vi "Three Button Dialog CORE.vi"(4 "Allow user to close window? (TRUE)":bool=TRUE, 5 "Justify Message (Left)":enum16{"Left", "Center", "Right"}(ring), 6 "Keyboard Shortcuts (Left is <Enter>)":T1={"Left Button Key Shortcut"={"Control"=FALSE, "Shift"=FALSE, "Key"="<Enter>"}, "Center Button Key Shortcut"={"Control"=FALSE, "Shift"=FALSE, "Key"=""}, "Right Button Key Shortcut"={"Control"=FALSE, "Shift"=FALSE, "Key"=""}}, 7 "Window Title (\"\")":string, 8 "Right Button Text (\"Cancel\")":string="Cancel", 9 "Center Button Text (\"No\")":string="No", 10 "Left Button Text (\"Yes\")":string="Yes", 11 "message":string) -> (3 "Which Button?":T2(ring)=enum."Center Button")   [LabVIEW 2011]
doc: "Displays text in a dialog with three buttons. The output enum indicates which of the three buttons the user chose, or it indicates that the user closed the dialog without making any choice."
panel:
  in  "OK":string="OK"
  out "C-Message":string
  in  "Right Button":bool
  in  "Center Button":bool
  in  "Left Button":bool
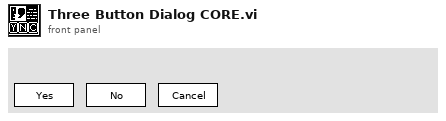
[diagram p1: front panel]
types:
  T1 = cluster{"Left Button Key Shortcut":cluster{"Control":bool, "Shift":bool, "Key":string}, "Center Button Key Shortcut":cluster{"Control":bool, "Shift":bool, "Key":string}, "Right Button Key Shortcut":cluster{"Control":bool, "Shift":bool, "Key":string}}
  T2 = enum16{"Left Button", "Center Button", "Right Button", "Window Close"}
  T3 = cluster{"left":i16, "top":i16, "right":i16, "bottom":i16}
  T4 = cluster{"Control":bool, "Shift":bool, "Key":string}
  T5 = cluster{bool, "Control":bool, "Shift":bool, "Key":string}
  T6 = typedef "LVRectTypeDef.ctl" = cluster{"left":i16, "top":i16, "right":i16, "bottom":i16}
  T7 = typedef "LVBoundsTypeDef.ctl" = cluster{"Width":u32, "Height":u32}
  T8 = typedef "LVPointTypeDef.ctl" = cluster{"Horizontal":i16, "Vertical":i16}
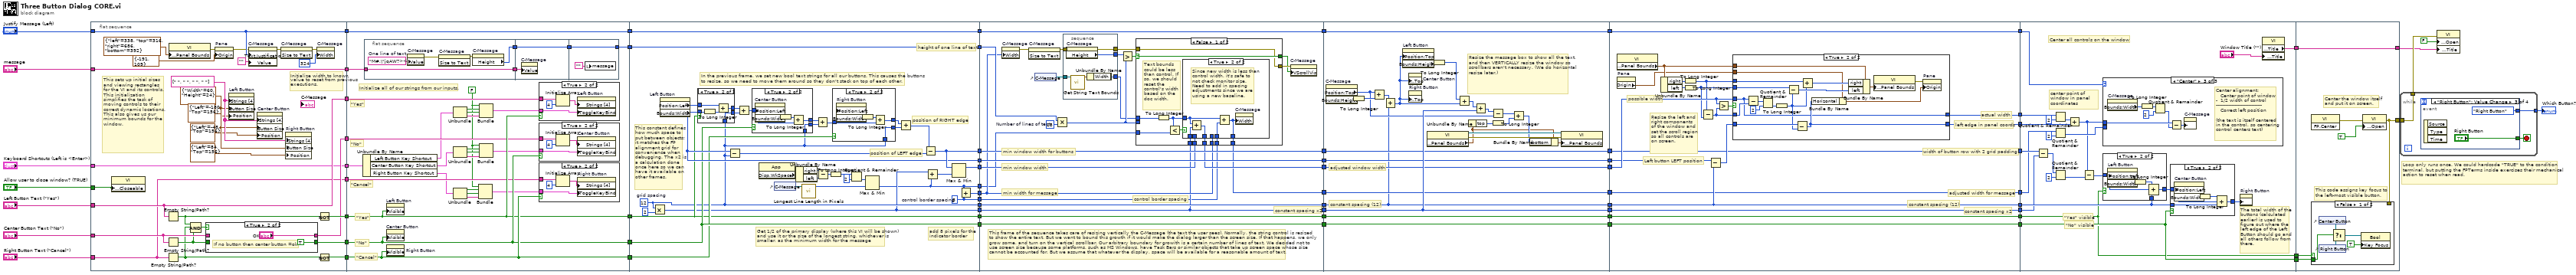
[diagram p0: block diagram]
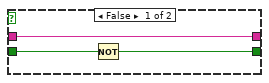
[diagram p2: hidden frame]
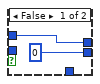
[diagram p6: hidden frame]
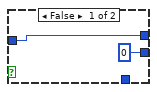
[diagram p7: hidden frame]
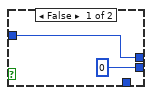
[diagram p8: hidden frame]
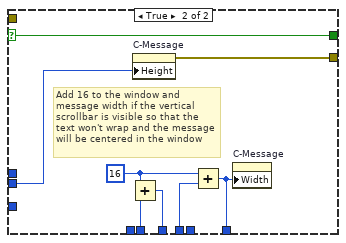
[diagram p10: hidden frame]
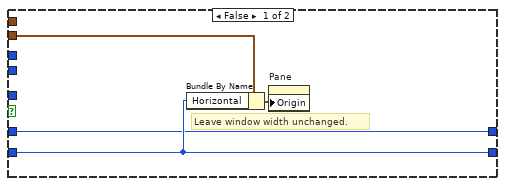
[diagram p11: hidden frame]
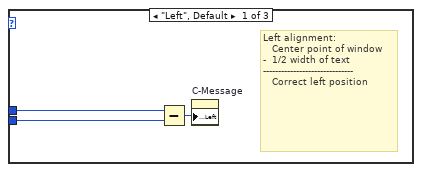
[diagram p12: hidden frame]
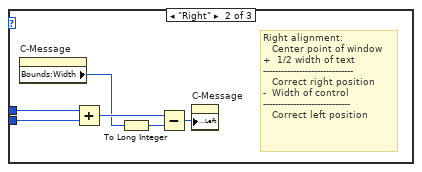
[diagram p13: hidden frame]
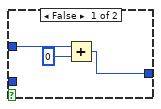
[diagram p14: hidden frame]
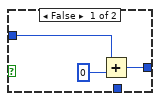
[diagram p15: hidden frame]
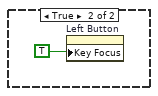
[diagram p16: hidden frame]
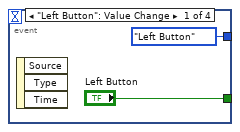
[diagram p17: hidden frame]
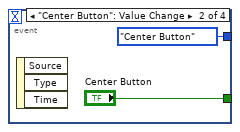
[diagram p18: hidden frame]
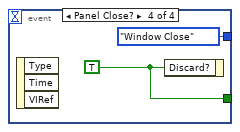
[diagram p19: hidden frame]
diagram:
  # "Loop only runs once. We could hardcode \"TRUE\" to the condition terminal, but putting the FPTerms inside exercises their mechanical action to reset when read."
  n1 = flat-sequence {
    tunnel: [w86] -> w14
    tunnel: [w88] -> w13
    tunnel: [w87] -> w12
    tunnel: [w82] -> w11
    tunnel: [w83] -> w10
    tunnel: [w80] -> w9
    tunnel: [w79] -> w8
    tunnel: "Left Button Text (\"Yes\")" -> [w82]
    tunnel: "Center Button Text (\"No\")" -> [w81]
    tunnel: "Right Button Text (\"Cancel\")" -> [w80]
    tunnel: "Justify Message (Left)" -> [w79]
    tunnel: "Keyboard Shortcuts (Left is <Enter>)" -> [w76]
    tunnel: [w76] -> w7
    tunnel: "message" -> [w75]
    tunnel: [w75] -> w6
    tunnel: "Allow user to close window? (TRUE)" -> [w74]
    tunnel: w14 -> [w130]
    tunnel: [w130] -> w64
    tunnel: w13 -> [w129]
    tunnel: [w129] -> w63
    tunnel: w12 -> [w128]
    tunnel: [w128] -> w62
    tunnel: w11 -> [w127]
    tunnel: w10 -> [w126]
    tunnel: w9 -> [w125]
    tunnel: w8 -> [w124]
    tunnel: [w124] -> w61
    tunnel: [w120] -> w60
    tunnel: w7 -> [w123]
    tunnel: w6 -> [w119]
    tunnel: [w185] -> w59
    tunnel: [w182] -> w58
    tunnel: [w181] -> w57
    tunnel: [w164] -> w56
    tunnel: [w163] -> w55
    tunnel: w64 -> [w174]
    tunnel: w63 -> [w176]
    tunnel: [w176] -> w54
    tunnel: w62 -> [w172]
    tunnel: [w172] -> w53
    tunnel: [w155] -> w52
    tunnel: w61 -> [w167]
    tunnel: [w167] -> w51
    tunnel: w60 -> [w166]
    tunnel: [w166] -> w50
    tunnel: [w153] -> w3
    tunnel: [w152] -> w2
    tunnel: w59 -> [w220]
    tunnel: [w219] -> w49
    tunnel: w58 -> [w226]
    tunnel: [w226] -> w48
    tunnel: w57 -> [w225]
    tunnel: [w225] -> w47
    tunnel: w56 -> [w224]
    tunnel: [w224] -> w46
    tunnel: w55 -> [w213]
    tunnel: [w213] -> w45
    tunnel: w54 -> [w223]
    tunnel: [w223] -> w44
    tunnel: w53 -> [w222]
    tunnel: [w222] -> w43
    tunnel: w52 -> [w214]
    tunnel: [w218] -> w42
    tunnel: w51 -> [w221]
    tunnel: [w221] -> w41
    tunnel: w50 -> [w216]
    tunnel: w3 -> [w212]
    tunnel: w2 -> [w211]
    tunnel: w49 -> [w275]
    tunnel: [w275] -> w40
    tunnel: w48 -> [w274]
    tunnel: [w274] -> w39
    tunnel: w47 -> [w273]
    tunnel: [w273] -> w38
    tunnel: w46 -> [w266]
    tunnel: [w266] -> w37
    tunnel: w45 -> [w283]
    tunnel: [w283] -> w36
    tunnel: w44 -> [w272]
    tunnel: [w272] -> w35
    tunnel: w43 -> [w271]
    tunnel: [w271] -> w34
    tunnel: w42 -> [w270]
    tunnel: [w270] -> w33
    tunnel: w41 -> [w269]
    tunnel: [w269] -> w32
    tunnel: w40 -> [w310]
    tunnel: [w305] -> w31
    tunnel: w39 -> [w298]
    tunnel: [w298] -> w30
    tunnel: w38 -> [w304]
    tunnel: w37 -> [w303]
    tunnel: [w303] -> w29
    tunnel: w36 -> [w297]
    tunnel: [w297] -> w28
    tunnel: [w301] -> w27
    tunnel: w35 -> [w296]
    tunnel: [w296] -> w26
    tunnel: w34 -> [w295]
    tunnel: [w295] -> w25
    tunnel: w33 -> [w292]
    tunnel: [w292] -> w24
    tunnel: w32 -> [w294]
    tunnel: [w294] -> w23
    tunnel: [w335] -> w22
    tunnel: w31 -> [w354]
    tunnel: w30 -> [w347]
    tunnel: w29 -> [w351]
    tunnel: w28 -> [w346]
    tunnel: w27 -> [w353]
    tunnel: w26 -> [w334]
    tunnel: w25 -> [w333]
    tunnel: w24 -> [w339]
    tunnel: w23 -> [w340]
    tunnel: [w334] -> w5
    tunnel: [w333] -> w4
    tunnel: [w388] -> w67
    tunnel: [w390] -> w65
    tunnel: w22 -> [w390]
    tunnel: w5 -> [w386]
    tunnel: w4 -> [w387]
    frame #0 {
      w96 = string[] [" ", " ", " ", " "] ("Strings [4]")
      w95 = cluster{"Width":u32, "Height":u32} {"Width"=60, "Height"=24} ("Button Size")
      # "Initialize width to known value to reset from previous executions."
      # "This sets up initial sizes and viewing rectangles\nfor the VI and its controls. This initialization\nsimplifies the task of moving controls to their\ncorrect dynamic locations. This also gives us our\nminimum bounds for the window."
      n2 = property class="VI"("Front Panel Window:Closeable"=w74) -> ()  [unwired: 2 in, 2 out]
      n3 = Empty String/Path?(string/path=w82) -> (empty?=w90:bool)
      n4 = Empty String/Path?(string/path=w81) -> (empty?=w78:bool)
      n5 = Empty String/Path?(string/path=w80) -> (empty?=w77:bool)
      n6 = property class="VI"("Front Panel Window:Panel Bounds"=T3 {"left"=338, "top"=316, "right"=686, "bottom"=392} ("Front Panel.PanelBounds")) -> (error out=w73:errorcluster)  [unwired: 2 in, 1 out]
      n7 = Compound Arithmetic op=AND(w90, w77, w78) -> (w89:bool)
      n8 = case shown="True" w89 {
        tunnel: w78 -> [w99 _]
        tunnel: [w98 TRUE] -> w88
        tunnel: w81 -> [w97 _]
        tunnel: [w97 "OK"] -> w83
        frame False {
          n9 = Not(x=w99) -> (.not. x?=w98:bool)
        }
        frame True {
          # "If no button then center button =ok"
        }
      }
      n10 = property on="Pane" class="Pane"(error in=w73, "Origin"=cluster{"Horizontal":i16, "Vertical":i16} {"Horizontal"=-191, "Vertical"=109} ("Front Panel.Origin")) -> (error out=w72:errorcluster)  [unwired: 1 in, 1 out]
      n11 = property on="Left Button" class="Bool"("Strings [4]"=w96, "Button Size"=w95, "Position"=cluster{"Left":i32, "Top":i32} {"Left"=-180, "Top"=156}) -> ()  [unwired: 2 in, 2 out]
      n12 = property on="C-Message" class="Str"(error in=w72, "Text.Justification"=w79, "Value"="") -> (error out=w91:errorcluster)  [unwired: 1 in, 1 out]
      n13 = property on="Center Button" class="Bool"("Strings [4]"=w96, "Button Size"=w95, "Position"=cluster{"Left":i32, "Top":i32} {"Left"=-48, "Top"=156}) -> ()  [unwired: 2 in, 2 out]
      n14 = invoke on="C-Message" class="Str" method="Size to Text"(error in=w91) -> (error out=w70:errorcluster)  [unwired: 2 in, 2 out]
      n15 = property on="Right Button" class="Bool"("Strings [4]"=w96, "Button Size"=w95, "Position"=cluster{"Left":i32, "Top":i32} {"Left"=84, "Top"=156}) -> ()  [unwired: 2 in, 2 out]
      n16 = property on="C-Message" class="Str"(error in=w70, "Width"=u32 324 ("Size:Width")) -> ()  [unwired: 1 in, 2 out]
      n17 = Not(x=w90) -> (.not. x?=w87:bool)
      n18 = Not(x=w77) -> (.not. x?=w86:bool)
    }
    frame #1 {
      w104 = FALSE
      # "\"Cancel\""
      # "\"No\""
      # "\"Yes\""
      # "\"Cancel\""
      # "\"No\""
      # "\"Yes\""
      # "Initialize all of our strings from our inputs."
      n19 = Unbundle By Name(w123) -> ("Left Button Key Shortcut"=w117:T4, "Center Button Key Shortcut"=w109:T4, "Right Button Key Shortcut"=w103:T4)
      n20 = flat-sequence {
        tunnel: [w132] -> w122
        tunnel: w119 -> [w131]
        tunnel: [w131] -> w118
        tunnel: w122 -> [w137]
        tunnel: [w137] -> w121
        tunnel: w118 -> [w136]
        tunnel: w121 -> [w138]
        tunnel: [w138] -> w120
        frame #0 {
          w135 = "M#,\"jqAW?><"  # One line of text
          n21 = property on="C-Message" class="Str"("Value"=w135) -> (error out=w133:errorcluster)  [unwired: 2 in, 1 out]
          n22 = invoke on="C-Message" class="Str" method="Size to Text"(error in=w133) -> (error out=w134:errorcluster)  [unwired: 2 in, 2 out]
          n23 = property on="C-Message" class="Str"(error in=w134) -> ("Height"=w132:u32)  [unwired: 1 in, 2 out]
        }
        frame #1 {
          n24 = property on="C-Message" class="Str"("Value"=w136) -> ()  [unwired: 2 in, 2 out]
        }
        frame #2 {
          n25 = local write "message"("") -> ()
        }
      }
      n26 = property on="Left Button" class="Bool"("Visible"=w128) -> ()  [unwired: 2 in, 2 out]
      n27 = property on="Center Button" class="Bool"("Visible"=w129) -> ()  [unwired: 2 in, 2 out]
      n28 = property on="Right Button" class="Bool"("Visible"=w130) -> ()  [unwired: 2 in, 2 out]
      n29 = Unbundle(w117) -> ("Control"=w116:bool, "Shift"=w115:bool, "Key"=w114:string)
      n30 = Unbundle(w109) -> ("Control"=w112:bool, "Shift"=w111:bool, "Key"=w110:string)
      n31 = Unbundle(w103) -> ("Control"=w107:bool, "Shift"=w106:bool, "Key"=w105:string)
      n32 = Bundle(w104, "Control"=w107, "Shift"=w106, "Key"=w105) -> (w102:T5)  [unwired: 1 out]
      n33 = Bundle(w104, "Control"=w116, "Shift"=w115, "Key"=w114) -> (w113:T5)  [unwired: 1 out]
      n34 = Bundle(w104, "Control"=w112, "Shift"=w111, "Key"=w110) -> (w108:T5)  [unwired: 1 out]
      n35 = case shown="True" w128 {
        tunnel: w127 -> [_ w149]
        tunnel: w113 -> [_ w148]
        frame False {
        }
        frame True {
          n36 = Initialize Array(w149, 4 ("dimension size")) -> (w151:string[])
          n37 = property on="Left Button" class="Bool"("Strings [4]"=w151, "ToggleKeyBind"=w148) -> ()  [unwired: 2 in, 2 out]
        }
      }
      n38 = case shown="True" w129 {
        tunnel: w108 -> [_ w145]
        tunnel: w126 -> [_ w144]
        frame False {
        }
        frame True {
          n39 = Initialize Array(w144, 4 ("dimension size")) -> (w147:string[])
          n40 = property on="Center Button" class="Bool"("Strings [4]"=w147, "ToggleKeyBind"=w145) -> ()  [unwired: 2 in, 2 out]
        }
      }
      n41 = case shown="True" w130 {
        tunnel: w102 -> [_ w141]
        tunnel: w125 -> [_ w140]
        frame False {
        }
        frame True {
          n42 = Initialize Array(w140, 4 ("dimension size")) -> (w143:string[])
          n43 = property on="Right Button" class="Bool"("Strings [4]"=w143, "ToggleKeyBind"=w141) -> ()  [unwired: 2 in, 2 out]
        }
      }
    }
    frame #2 {
      w153 = 8  # control border spacing
      w164 = 12  # grid spacing
      # "position of RIGHT edge"
      # "height of one line of text"
      # "add 8 pixels for the indicator border"
      # "Get 1/2 of the primary display (where this VI will be shown) and use it or the size of the longest string, whichever is smaller, as the minimum width for the message"
      # "This constant defines how much space to put between objects; it matches the FP alignment grid for convenience when debugging. The x2 is a calculation done once here so we can have it available on other frames."
      # "In the previous frame, we set new bool text strings for all our buttons. This causes the buttons to resize, so we need to move them around so they don't stack on top of each other."
      # "position of LEFT edge"
      n44 = Multiply(x=w164, y=2) -> (x*y=w163:i32)
      n45 = property on="Left Button" class="Bool"() -> ("Position:Left"=w181:i32, "Bounds:Width"=w178:u32)  [unwired: 2 in, 2 out]
      n46 = case shown="True" w172 {
        tunnel: w181 -> [w188 w193]
        tunnel: w178 -> [_ w192]
        tunnel: [w188 w191] -> w173
        tunnel: w164 -> [_ w189]
        tunnel: [0 w189] -> w171
        frame False {
        }
        frame True {
          n47 = To Long Integer(number=w192) -> (32bit integer=w190:i32)
          n48 = Add(x=w193, y=w190) -> (x+y=w191:i32)
        }
      }
      n49 = Subtract(x=w181, y=w164) -> (x-y=w183:i32)
      n50 = Add(x=w173, y=w171) -> (x+y=w179:i32)
      n51 = case shown="True" w176 {
        tunnel: w179 -> [w202 w207]
        tunnel: [w202 w206] -> w177
        tunnel: [0 w203] -> w170
        tunnel: w164 -> [_ w203]
        frame False {
        }
        frame True {
          n52 = property on="Center Button" class="Bool"("Position:Left"=w207) -> ("Bounds:Width"=w205:u32)  [unwired: 2 in, 2 out]
          n53 = To Long Integer(number=w205) -> (32bit integer=w204:i32)
          n54 = Add(x=w204, y=w207) -> (x+y=w206:i32)
        }
      }
      n55 = property class="App"() -> ("Disp.WkSpace"=w162:T6)  [unwired: 2 in, 2 out]
      n56 = control-ref of="C-Message"() -> (w168:refnum<vi>)
      n57 = Unbundle By Name(w162) -> ("right"=w158:i16, "left"=w157:i16)
      n58 = call "Longest Line Length in Pixels.vi"("String"=w168) -> ("longest line length"=w159:i32)  [unwired: 1 in, 8 out]
      n59 = Add(x=w177, y=w170) -> (x+y=w180:i32)
      n60 = Subtract(x=w158, y=w157) -> (x-y=w161:i16)
      n61 = To Long Integer(number=w161) -> (32bit integer=w156:i32)
      n62 = case shown="True" w174 {
        tunnel: w180 -> [w195 w200]
        tunnel: [w195 w196] -> w175
        tunnel: [0 w197] -> w169
        tunnel: w164 -> [_ w197]
        frame False {
        }
        frame True {
          n63 = property on="Right Button" class="Bool"("Position:Left"=w200) -> ("Bounds:Width"=w199:u32)  [unwired: 2 in, 2 out]
          n64 = To Long Integer(number=w199) -> (32bit integer=w198:i32)
          n65 = Add(x=w198, y=w200) -> (x+y=w196:i32)
        }
      }
      n66 = Quotient & Remainder(x=w156, y=2) -> (floor(x/y)=w154:i32)  [unwired: 1 out]
      n67 = Max & Min(x=w154, y=w159) -> (min(x,y)=w152:i32)  [unwired: 1 out]
      n68 = Add(x=w175, y=w169) -> (x+y=w184:i32)
      n69 = Subtract(x=w184, y=w183) -> (x-y=w182:i32)
      n70 = Add(x=w163, y=w152) -> (x+y=w186:i32)
      n71 = Max & Min(x=w182, y=w186) -> (max(x,y)=w185:i32)  [unwired: 1 out]
      n72 = Add(x=w152, y=w153) -> (x+y=w155:i32)
    }
    frame #3 {
      w228 = u32 25  # Number of lines of text
      # "control border spacing"
      # "constant spacing x2"
      # "min window width for buttons"
      # "min window width"
      # "min width for message"
      # "This frame of the sequence takes care of resizing vertically the C-Message (the text the user sees). Normally, the string control is resized to show the entire text. But we want to bound this growth if it would make the dialog larger than the screen size. If that happens, we only grow some, and turn on the vertical scrollbar. Our arbitrary boundary for growith is a certain number of lines of text. We decided not to use screen size because some platforms, such as MS Windows, have Task Bars or similar objects that take up screen space whose size cannot be accounted for. But we assume that whatever the display, space will be available for a reasonable amount of text."
      n73 = property on="C-Message" class="Str"("Width"=w214) -> (error out=w217:errorcluster)  [unwired: 2 in, 1 out]
      n74 = invoke on="C-Message" class="Str" method="Size to Text"(error in=w217) -> (error out=w232:errorcluster)  [unwired: 2 in, 2 out]
      n75 = control-ref of="C-Message"() -> (w209:refnum<vi>)
      n76 = Multiply(x=w216, y=w228) -> (x*y=w227:u32)
      n77 = stacked-sequence {
        tunnel: w232 -> [w238]
        tunnel: [w237] -> w215
        tunnel: [w236] -> w210
        tunnel: w209 -> [w235]
        tunnel: [w233] -> w208
        frame #0 {
          n78 = property on="C-Message" class="Str"(error in=w238) -> (error out=w236:errorcluster, "Height"=w237:u32)  [unwired: 1 in, 1 out]
          n79 = call "Get String Text Bounds.vi"("String"=w235) -> ("Text bounds"=w234:T7)  [unwired: 10 out]
          n80 = Unbundle By Name(w234) -> ("Width"=w233:u32)
        }
      }
      n81 = Greater?(x=w215, y=w227) -> (0:w231:bool)
      n82 = case shown="False" w231 {
        selector: w231 -> [w250 w264]
        tunnel: [w249 w265] -> w230
        tunnel: [w250 w264] -> w229
        tunnel: w210 -> [w249 _]
        tunnel: w227 -> [_ w263]
        tunnel: [w243 w261] -> w219
        tunnel: w220 -> [w245 w262]
        tunnel: [w242 w258] -> w218
        tunnel: w214 -> [w244 w260]
        tunnel: w208 -> [w247 _]
        tunnel: w211 -> [w246 _]
        tunnel: w213 -> [w241 _]
        tunnel: w212 -> [w240 _]
        frame False {
          # "Text bounds could be less than control. If so, we should reset the control's width based on the doc width."
          n83 = To Long Integer(number=w247) -> (32bit integer=w239:i32)
          n84 = Less?(x=w239, y=w246) -> (x < y?=w248:bool)
          n85 = case shown="True" w248 {
            tunnel: w239 -> [_ w256]
            tunnel: w245 -> [w252 _]
            tunnel: w244 -> [w251 _]
            tunnel: [w252 w255] -> w243
            tunnel: [w251 w254] -> w242
            tunnel: w241 -> [_ w257]
            tunnel: w240 -> [_ w253]
            frame False {
            }
            frame True {
              # "Since new width is less than control width, it's safe to not check monitor size. \nNeed to add in spacing adjustments since we are using a new baseline."
              n86 = Add(x=w256, y=w257) -> (x+y=w255:i32)
              n87 = Add(x=w256, y=w253) -> (x+y=w254:i32)
              n88 = property on="C-Message" class="Str"("Width"=w254) -> ()  [unwired: 2 in, 2 out]
            }
          }
        }
        frame True {
          w259 = 16 ("x")
          # "Add 16 to the window and message width if the vertical scrollbar is visible so that the text won't wrap and the message will be centered in the window"
          n89 = Add(x=w259, y=w262) -> (x+y=w261:i32)
          n90 = property on="C-Message" class="Str"("Height"=w263) -> (error out=w265:errorcluster)  [unwired: 2 in, 1 out]
          n91 = Add(x=w259, y=w260) -> (x+y=w258:i32)
          n92 = property on="C-Message" class="Str"("Width"=w258) -> ()  [unwired: 2 in, 2 out]
        }
      }
      n93 = property on="C-Message" class="Str"(error in=w230, "VScrollVis"=w229) -> ()  [unwired: 1 in, 2 out]
    }
    frame #4 {
      # "adjusted window width"
      # "constant spacing (12)"
      # "Resize the message box to show all the text, and then VERTICALLY resize the window so scrollbars aren't necessary. (We do horizontal resize later.)"
      n94 = property on="C-Message" class="Str"() -> ("Position:Top"=w277:i32, "Bounds:Height"=w276:u32)  [unwired: 2 in, 2 out]
      n95 = To Long Integer(number=w276) -> (32bit integer=w282:i32)
      n96 = Add(x=w277, y=w282) -> (x+y=w267:i32)
      n97 = Add(x=w267, y=w266) -> (x+y=w268:i32)
      n98 = property on="Left Button" class="Bool"("Position:Top"=w268) -> ("Bounds:Height"=w279:u32)  [unwired: 2 in, 2 out]
      n99 = property on="Center Button" class="Bool"("Position:Top"=w268) -> ()  [unwired: 2 in, 2 out]
      n100 = property on="Right Button" class="Bool"("Position:Top"=w268) -> ()  [unwired: 2 in, 2 out]
      n101 = property class="VI"() -> (reference out=w289:refnum<vi>, error out=w290:errorcluster, "Front Panel Window:Panel Bounds"=w280:T6)  [unwired: 2 in]
      n102 = To Long Integer(number=w279) -> (32bit integer=w278:i32)
      n103 = Add(x=w278, y=w268) -> (x+y=w284:i32)
      n104 = Unbundle By Name(w280) -> ("top"=w287:i16)
      n105 = Add(x=w284, y=w283) -> (x+y=w285:i32)
      n106 = Subtract(x=w285, y=w277) -> (x-y=w288:i32)
      n107 = To Long Integer(number=w287) -> (32bit integer=w281:i32)
      n108 = Add(x=w288, y=w281) -> (x+y=w286:i32)
      n109 = Bundle By Name(cluster=w280, "bottom"=w286) -> (w291:T6)
      n110 = property class="VI"(reference=w289, error in=w290, "Front Panel Window:Panel Bounds"=w291) -> ()  [unwired: 2 out]
    }
    frame #5 {
      # "adjusted width for message"
      # "constant spacing x2"
      # "constant spacing (12)"
      # "Left button LEFT position"
      # "left edge in panel coords"
      # "width of button row with 2 grid padding"
      # "Resize the left and\nright components\nof the window and\nset the scroll region\nso all controls are \non screen."
      # "actual width"
      # "possible width"
      n111 = property class="VI"() -> ("Front Panel Window:Panel Bounds"=w307:T6)  [unwired: 2 in, 2 out]
      n112 = property on="Pane" class="Pane"() -> ("Origin"=w293:T8)  [unwired: 2 in, 2 out]
      n113 = Unbundle By Name(w307) -> ("right"=w309:i16, "left"=w308:i16)
      n114 = To Long Integer(number=w309) -> (32bit integer=w299:i32)
      n115 = To Long Integer(number=w308) -> (32bit integer=w300:i32)
      n116 = Subtract(x=w299, y=w300) -> (x-y=w311:i32)
      n117 = Subtract(x=w304, y=w303) -> (x-y=w302:i32)
      n118 = Greater?(x=w310, y=w311) -> (0:w306:bool)
      n119 = case shown="True" w306 {
        tunnel: w311 -> [w313 w332]
        tunnel: w310 -> [_ w319]
        tunnel: w299 -> [_ w327]
        tunnel: w300 -> [_ w328]
        tunnel: w307 -> [_ w329]
        tunnel: [w315 w321] -> w305
        tunnel: w293 -> [w314 w322]
        tunnel: w302 -> [w315 w320]
        tunnel: [w313 w319] -> w301
        frame False {
          # "Leave window width unchanged."
          n120 = Bundle By Name(cluster=w314, "Horizontal"=w315) -> (w312:T8)
          n121 = property on="Pane" class="Pane"("Origin"=w312) -> ()  [unwired: 2 in, 2 out]
        }
        frame True {
          n122 = Subtract(x=w319, y=w332) -> (x-y=w331:i32)
          n123 = Quotient & Remainder(x=w331, y=2) -> (floor(x/y)=w324:i32)  [unwired: 1 out]
          n124 = To Long Integer(number=w324) -> (32bit integer=w318:i32)
          n125 = Subtract(x=w328, y=w318) -> (x-y=w325:i32)
          n126 = Subtract(x=w320, y=w318) -> (x-y=w321:i32)
          n127 = Add(x=w327, y=w318) -> (x+y=w326:i32)
          n128 = Bundle By Name(cluster=w322, "Horizontal"=w321) -> (w316:T8)
          n129 = Bundle By Name(cluster=w329, "right"=w326, "left"=w325) -> (w323:T6)
          n130 = property class="VI"("Front Panel Window:Panel Bounds"=w323) -> (error out=w317:errorcluster)  [unwired: 2 in, 1 out]
          n131 = property on="Pane" class="Pane"(error in=w317, "Origin"=w316) -> ()  [unwired: 1 in, 2 out]
        }
      }
    }
    frame #6 {
      # "\"No\" visible"
      # "\"Yes\" visible"
      # "The total width of the buttons (calculated earlier) is used to figure out where the left edge of the Left Button should go and all others follow from there."
      # "center point of window in panel coordinates"
      # "Center all controls on the window"
      n132 = Subtract(x=w347, y=w346) -> (x-y=w348:i32)
      n133 = Quotient & Remainder(x=w353, y=2) -> (floor(x/y)=w350:i32)  [unwired: 1 out]
      n134 = Quotient & Remainder(x=w339, y=2) -> (floor(x/y)=w338:i32)  [unwired: 1 out]
      n135 = Quotient & Remainder(x=w348, y=2) -> (floor(x/y)=w345:i32)  [unwired: 1 out]
      n136 = Add(x=w350, y=w354) -> (x+y=w337:i32)
      n137 = Subtract(x=w337, y=w345) -> (x-y=w344:i32)
      n138 = case shown="\"Center\"" w340 {
        tunnel: w337 -> [w357 w363 w365]
        tunnel: w338 -> [w355 w362 _]
        frame "Left", Default {
          # "Left alignment:\n   Center point of window\n-  1/2 width of text\n------------------------------\n   Correct left position"
          n139 = Subtract(x=w357, y=w355) -> (x-y=w356:i32)
          n140 = property on="C-Message" class="Str"("Position:Left"=w356) -> ()  [unwired: 2 in, 2 out]
        }
        frame "Right" {
          # "Right alignment:\n   Center point of window\n+  1/2 width of text\n------------------------------\n   Correct right position\n-  Width of control\n-----------------------------\n   Correct left position"
          n141 = property on="C-Message" class="Str"() -> ("Bounds:Width"=w359:u32)  [unwired: 2 in, 2 out]
          n142 = Add(x=w363, y=w362) -> (x+y=w361:i32)
          n143 = To Long Integer(number=w359) -> (32bit integer=w358:i32)
          n144 = Subtract(x=w361, y=w358) -> (x-y=w360:i32)
          n145 = property on="C-Message" class="Str"("Position:Left"=w360) -> ()  [unwired: 2 in, 2 out]
        }
        frame "Center" {
          # "Center alignment:\n   Center point of window\n-  1/2 width of control\n------------------------------\n   Correct left position\n\n(the text is itself centered in the control, so centering control centers text)"
          n146 = property on="C-Message" class="Str"() -> ("Bounds:Width"=w368:u32)  [unwired: 2 in, 2 out]
          n147 = To Long Integer(number=w368) -> (32bit integer=w366:i32)
          n148 = Quotient & Remainder(x=w366, y=2) -> (floor(x/y)=w364:i32)  [unwired: 1 out]
          n149 = Subtract(x=w365, y=w364) -> (x-y=w367:i32)
          n150 = property on="C-Message" class="Str"("Position:Left"=w367) -> ()  [unwired: 2 in, 2 out]
        }
      }
      n151 = case shown="True" w333 {
        tunnel: w351 -> [_ w385]
        tunnel: w344 -> [w380 w384]
        tunnel: [w379 w382] -> w343
        frame False {
          n152 = Add(x=w380, y=0) -> (x+y=w379:i32)
        }
        frame True {
          n153 = property on="Left Button" class="Bool"("Position:Left"=w384) -> ("Bounds:Width"=w383:u32)  [unwired: 2 in, 2 out]
          n154 = To Long Integer(number=w383) -> (32bit integer=w381:i32)
          n155 = Compound Arithmetic op=ADD(w381, w384, w385) -> (w382:i32)
        }
      }
      n156 = case shown="True" w334 {
        tunnel: w351 -> [_ w377]
        tunnel: w343 -> [w372 w375]
        tunnel: [w371 w374] -> w342
        frame False {
          n157 = Add(x=w372, y=0) -> (x+y=w371:i32)
        }
        frame True {
          n158 = property on="Center Button" class="Bool"("Position:Left"=w375) -> ("Bounds:Width"=w376:u32)  [unwired: 2 in, 2 out]
          n159 = To Long Integer(number=w376) -> (32bit integer=w373:i32)
          n160 = Compound Arithmetic op=ADD(w373, w375, w377) -> (w374:i32)
        }
      }
      n161 = property on="Right Button" class="Bool"("Position:Left"=w342) -> ()  [unwired: 2 in, 2 out]
      n162 = property class="VI"("Front Panel Window:Title"="Window Title (\"\")") -> ("Front Panel Window:Title"=w335:string)  [unwired: 2 in, 2 out]
    }
    frame #7 {
      # "This code assigns key focus to\nthe left-most visible button."
      # "Center the window itself and put it on screen."
      n163 = invoke class="VI" method="FP.Center"() -> (error out=w389:errorcluster)  [unwired: 3 in, 2 out]
      n164 = property class="VI"(error in=w389, "Front Panel Window:Open"=TRUE) -> (error out=w388:errorcluster)  [unwired: 1 in, 1 out]
      n165 = case shown="False" w387 {
        tunnel: w388 -> [_ _]
        tunnel: w386 -> [w396 _]
        frame False {
          n166 = control-ref of="Center Button"() -> (w395:refnum<vi>)
          n167 = control-ref of="Right Button"() -> (w394:refnum<vi>)
          n168 = Select(t=w395, s=w396, f=w394) -> (s? t:f=w393:refnum<vi>)
          n169 = property class="Bool"(reference=w393, "Key Focus"=TRUE) -> ()  [unwired: 1 in, 2 out]
        }
        frame True {
          n170 = property on="Left Button" class="Bool"("Key Focus"=TRUE) -> ()  [unwired: 2 in, 2 out]
        }
      }
    }
  }
  n171 = while {
    tunnel: [w400] -> w68
    tunnel: [w399] -> w66
    tunnel: w67 -> [w399]
    stop <- w398 stop-if-true
    n172 = event shown="[2] \"Right Button\": Value Change" {
      selector: _ -> [_ _ _ _]
      dyn-events: _ -> [_ _ _ _]
      timeout: _ -> [_ _ _ _]
      tunnel: ["Left Button" "Center Button" "Right Button" w407] -> w398
      tunnel: [T2."Left Button" ("Which Button?") T2."Center Button" ("Which Button?") T2."Right Button" ("Which Button?") T2."Window Close" ("Which Button?")] -> w400
      event "Left Button": Value Change {
        n173 = event-data() -> ()  [unwired: 4 out]
      }
      event "Center Button": Value Change {
        n174 = event-data() -> ()  [unwired: 4 out]
      }
      event "Right Button": Value Change {
        n175 = event-data() -> ()  [unwired: 4 out]
      }
      event Panel Close? {
        w407 = TRUE ("Discard?")
        n176 = event-data() -> ()  [unwired: 4 out]
        n177 = event-data("Discard?"=w407) -> ()  [unwired: 1 in, 1 out]
      }
    }
  }
  "Which Button?" <- w68
  n178 = property class="VI"(error in=w66, "Front Panel Window:Open"=FALSE, "Front Panel Window:Title"=w65) -> ()  [unwired: 1 in, 2 out]
